vi "UpperCase.vi"() -> ()   [LabVIEW 2015]
panel:
  out "String 2":string
  in  "String":string
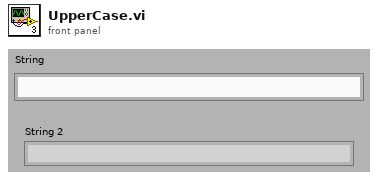
[diagram p1: front panel]
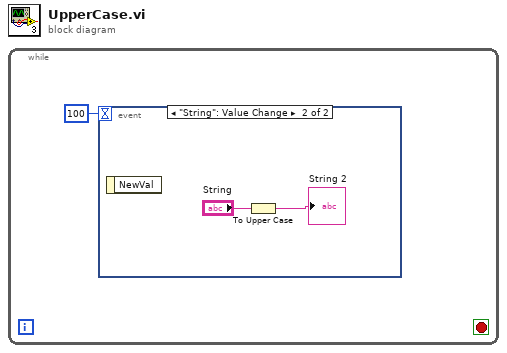
[diagram p0: block diagram]
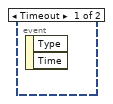
[diagram p2: hidden frame]
diagram:
  n1 = while {
    stop <- _ stop-if-true
    n2 = event shown="[1] \"String\": Value Change" {
      selector: _ -> [_ _]
      dyn-events: _ -> [_ _]
      timeout: 100 -> [_ _]
      event Timeout {
        n3 = event-data() -> ()  [unwired: 1 in, 2 out]
      }
      event "String": Value Change {
        n4 = event-data() -> ()  [unwired: 1 in, 1 out]
        n5 = To Upper Case(1:"String") -> (0:→"String 2":string)
      }
    }
  }
